vi "InitAction.vi"(6 "InstrumentName":string, 7 "VisaRessIn":refnum<visa-resource-name>, 8 "error in (no error)":errorcluster caption="entrée d'erreur (pas d'erreur)", 9 "FirstClassInst":bool, 10 "Function":string, 11 "GenData In":refnum<class "ThorPM100A.lvclass"> caption="DNL_LabVIEW Object in") -> (0 "error out":errorcluster caption="sortie d'erreur", 3 "GenData Out":refnum<class "ThorPM100A.lvclass"> caption="DNL_LabVIEW Object out")   [LabVIEW 2019, in "ThorPM100A.lvclass"]
uses:
  ThorPM100A.lvclass
  C:/Programmes Labview/LabScanV1A/DevicesClass/BaseDevice/BaseDevice.lvclass
  ThorPM100A_Func.ctl
  ThorPM100A.lvclass/ThorPM100A.ctl
  <vilib>/Utility/error.llb/Error Cluster From Error Code.vi
  <vilib>/ErrorRing/Error Ring.xnode
panel:
  out "Device Available":bool
  in  "DefaultDev_Func":T1
  out "VisaRessOut":refnum<visa-resource-name>
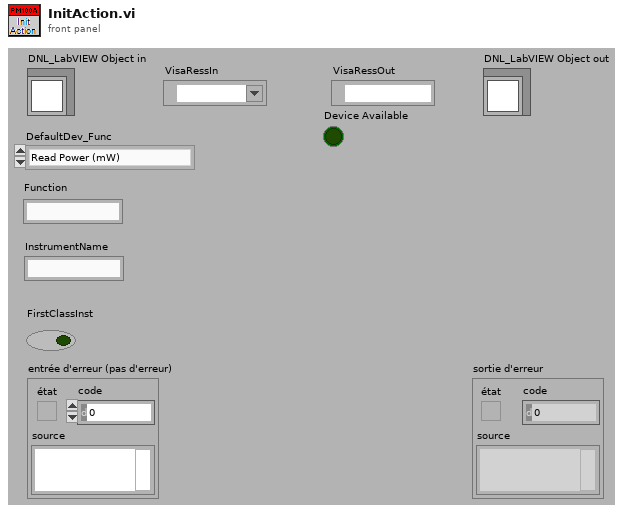
[diagram p1: front panel]
types:
  T1 = typedef "ThorPM100A.lvclass/ThorPM100A_Func.ctl" = enum16{"Read Power (mW)"}
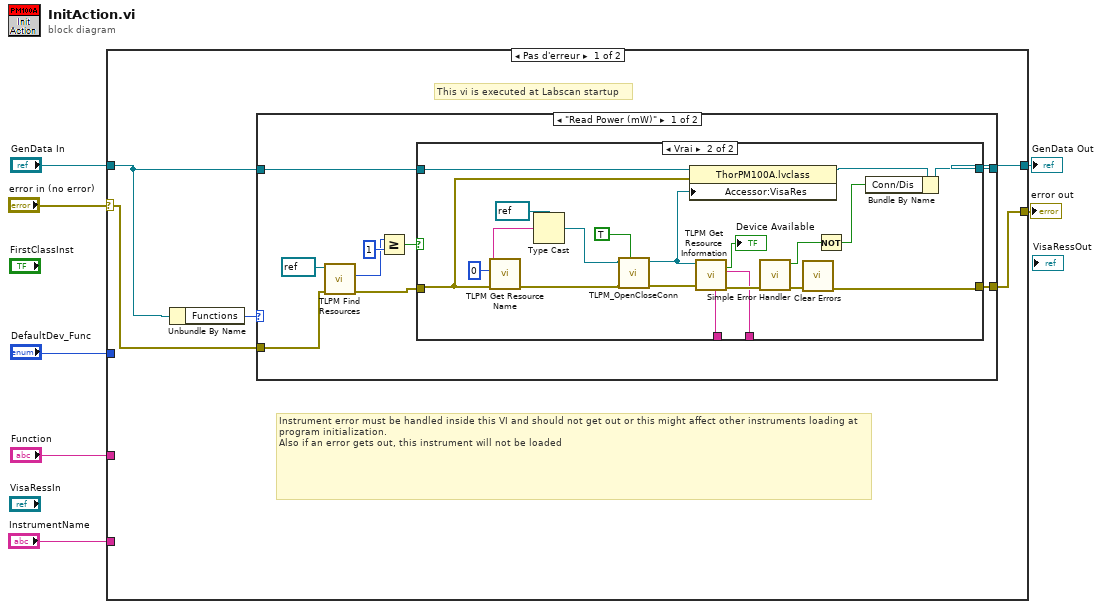
[diagram p0: block diagram]
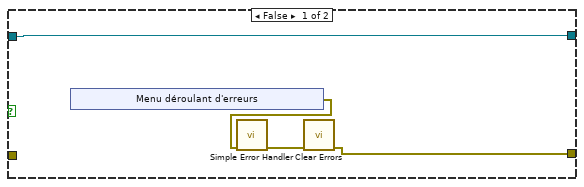
[diagram p2: hidden frame]
diagram:
  n1 = case shown="Pas d'erreur" "error in (no error)" {
    selector: "error in (no error)" -> [w9 w54]
    tunnel: [w8 w54] -> w6
    tunnel: "GenData In" -> [w10 w53]
    tunnel: [w11 w53] -> w4
    tunnel: "DefaultDev_Func" -> [_ _]
    tunnel: "Function" -> [_ _]
    tunnel: "InstrumentName" -> [_ _]
    frame No Error {
      # "This vi is executed at Labscan startup"
      # "Instrument error must be handled inside this VI and should not get out or this might affect other instruments loading at program initialization.\nAlso if an error gets out, this instrument will not be loaded"
      n2 = Unbundle By Name(w10) -> ("Functions"=w12:T1)
      n3 = case shown="\"Read Power (mW)\"" w12 {
        tunnel: [w20 w52] -> w11
        tunnel: w10 -> [w21 w52]
        tunnel: w9 -> [w14 w51]
        tunnel: [w19 w51] -> w8
        frame "Read Power (mW)" {
          n4 = call <instrlib>:"TLPM Find Resources.vi"("error in (no error)"=w14, "instrument handle"=refnum<visa-resource-name> refnum) -> ("error out"=w13:errorcluster, "Resource Count"=w15:u32)  [unwired: 7 in, 1 out]
          n5 = Greater Or Equal?(x=w15, y=u32 1) -> (x >= y?=w16:bool)
          n6 = case shown="Vrai" w16 {
            tunnel: w21 -> [w25 w49]
            tunnel: [w25 w33] -> w20
            tunnel: [w22 w46] -> w19
            tunnel: w13 -> [_ w47]
            tunnel: [_ w43] -> _
            tunnel: [_ w42] -> _
            frame False {
              n7 = xnode "Menu déroulant d'erreurs"() -> ("sortie d'erreur"=w23:errorcluster)
              n8 = call <vilib>:"Simple Error Handler.vi"("error in (no error)"=w23) -> ("error out"=w24:errorcluster)  [unwired: 4 in, 4 out]
              n9 = call <vilib>:"Clear Errors.vi"("error in (no error)"=w24) -> ("error out"=w22:errorcluster)  [unwired: 5 in, 1 out]
            }
            frame True {
              n10 = call <instrlib>:"TLPM Get Resource Name.vi"("error in (no error)"=w47, "Index (0)"=u32 0 ("Device Index")) -> ("error out"=w36:errorcluster, "Resource Name"=w39:string)  [unwired: 7 in, 1 out]
              n11 = Type Cast(type=refnum<visa-resource-name> refnum ("VISA resource name"), x=w39) -> (*(type *) &x=w37:refnum<visa-resource-name>)
              n12 = call <instrlib>:"TLPM_OpenCloseConn.vi"("Open"=TRUE, "error in"=w36, "ConnID"=w37) -> ("error out"=w35:errorcluster, "connection ID"=w38:refnum<visa-resource-name>)  [unwired: 7 in]
              n13 = property class="ThorPM100A.lvclass"(reference=w49, error in=w47, "Accessor:VisaRes"=w38) -> (reference out=w48:refnum<class "ThorPM100A.lvclass">)  [unwired: 1 out]
              n14 = call <instrlib>:"TLPM Get Resource Information.vi"("error in (no error)"=w35, "instrument handle"=w38) -> ("error out"=w45:errorcluster, "Model Name"=w42:string, "Manufacturer"=w43:string, "Device Available"=→"Device Available":bool)  [unwired: 4 in, 2 out]
              n15 = call <vilib>:"Simple Error Handler.vi"("error in (no error)"=w45) -> ("error?"=w32:bool, "error out"=w44:errorcluster)  [unwired: 4 in, 3 out]
              n16 = call <vilib>:"Clear Errors.vi"("error in (no error)"=w44) -> ("error out"=w46:errorcluster)  [unwired: 5 in, 1 out]
              n17 = Not(x=w32) -> (.not. x?=w31:bool)
              n18 = Bundle By Name(cluster=w48, "Conn/Dis"=w31) -> (w33:refnum<class "ThorPM100A.lvclass">)
            }
          }
        }
        frame Default {
        }
      }
    }
    frame Error {
    }
  }
  "error out" <- w6
  "GenData Out" <- w4
